vi "FTW-Container-QueryValueByPath.vi"(0 "Container":refnum<class "FTW-Container.lvclass">, 5 "Type and Defaults":variant, 7 "Query":string, 11 "error in":errorcluster) -> (4 "Container out":refnum<class "FTW-Container.lvclass">, 6 "Result":variant, 15 "error out":errorcluster)   [LabVIEW 2012, in "FTW-Container.lvclass"]
uses:
  FTW-Container.lvclass
panel:
  # "Inputs"
  # "Outputs"
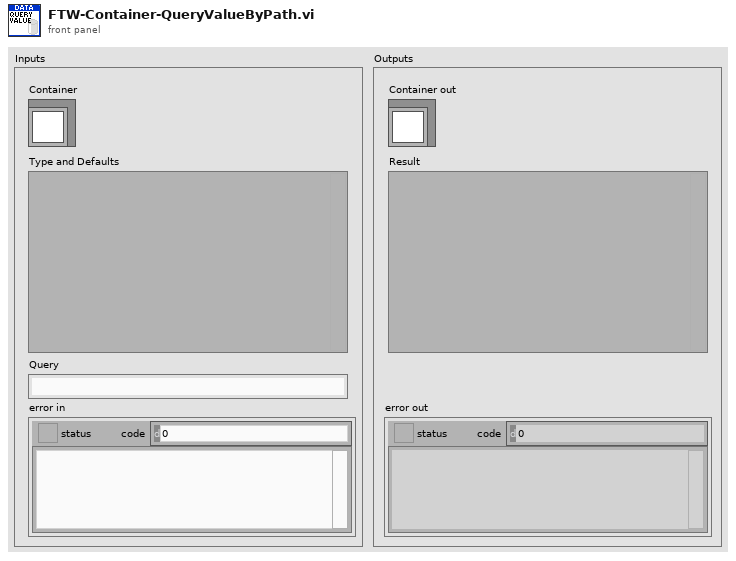
[diagram p1: front panel]
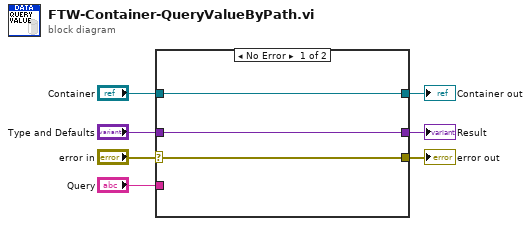
[diagram p0: block diagram]
diagram:
  n1 = case shown="No Error" "error in" {
    selector: "error in" -> [w8 w13]
    tunnel: [w8 w13] -> w7
    tunnel: "Container" -> [w10 w12]
    tunnel: [w10 w12] -> w4
    tunnel: "Type and Defaults" -> [w9 w11]
    tunnel: [w9 w11] -> w2
    tunnel: "Query" -> [_ _]
    frame No Error {
    }
    frame Error {
    }
  }
  "error out" <- w7
  "Container out" <- w4
  "Result" <- w2
